vi "oax_gsOverview.vi"() -> ()   [LabVIEW 2017]
panel:
  in  "String":string="       Getting Started with Gabor Order Tracking Demo Overview\n\nThe NI Sound and Vibration Measurement Suite provides Order Analysis VIs for analyzing sound or vibration signals generated by rotating or reciprocating machinery, such as engines, compressors, turbines, and pumps. With the Order Analysis VIs, you can reduce sound or vibration signals to meaningful formats, separate rotational and structural components, associate signal components with specific mechanical parts, and perform repeatable measurements. You mainly use Order Analysis VIs in noise, vibration and harshness (NVH) testing as well as machine condition monitoring (MCM) applications.\n\nThe Getting Started with Gabor Order Tracking VI uses Gabor transform method to extract order-related information. This VI includes three basic functions to perform order analysis: Data Logger, Tacho Analyzer, and Order Analyzer. \n\nYou can use the Data Logger to acquire and log to disk a sound or vibration signal and a tachometer signal. \n\nIn Tacho Analyzer, you can load the acquired sound or vibration signal and the tachometer signal into the Getting Started with Gabor Order Tracking VI separately. You can perform signal conditioning on the tachometer signal. You then can save the sound or vibration signal and the conditioned tachometer signal in one file for further analysis.\n\nWith the Order Analyzer, you can view the sound or vibration signal in colormap with different plot type, such as frequency-time, frequency-RPM, or order-RPM. You also can extract time waveforms of specified orders in this VI. After you extract the time waveform of a specific order, you can use the sound playback function to playback the sound of that particular order.\n"
  in  "STOP":bool
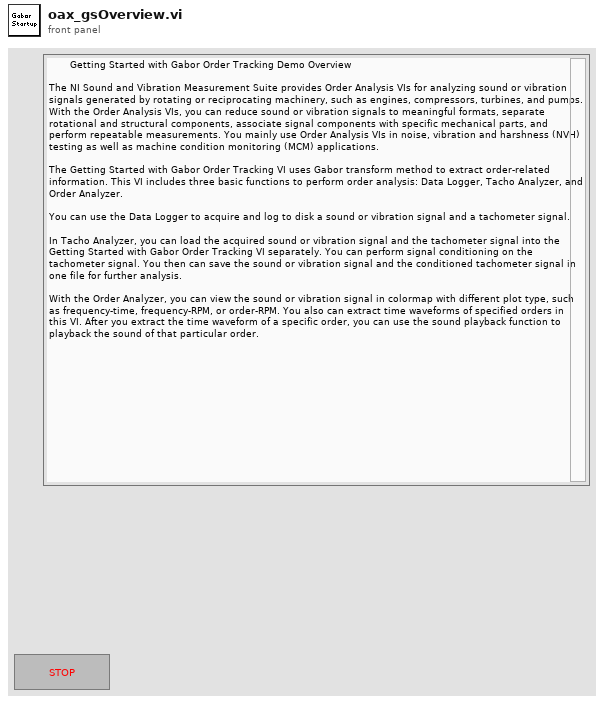
[diagram p1: front panel]
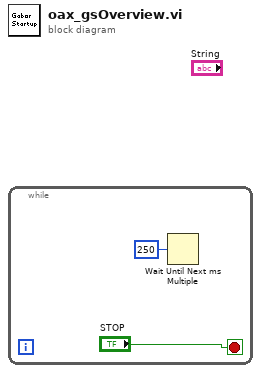
[diagram p0: block diagram]
diagram:
  n1 = while {
    stop <- "STOP" stop-if-true
    n2 = Wait Until Next ms Multiple(millisecond multiple=u32 250) -> ()  [unwired: 1 out]
  }
